vi "Relink Renamed Files to Library.vi"(8 "error in":errorcluster, 10 "plugin library path":path, 11 "plugin files path":path[](array[path])) -> (0 "error out":errorcluster)   [LabVIEW 2021, in "InstrumentStudio Plug-In Editor.lvlib"]
uses:
  InstrumentStudio Plug-In Editor.lvlib
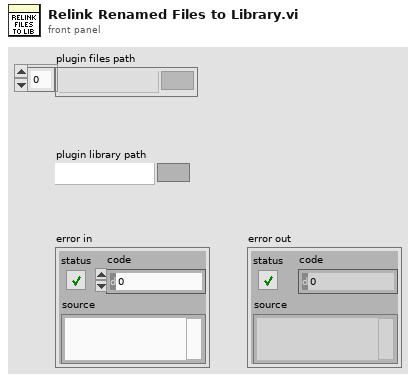
[diagram p1: front panel]
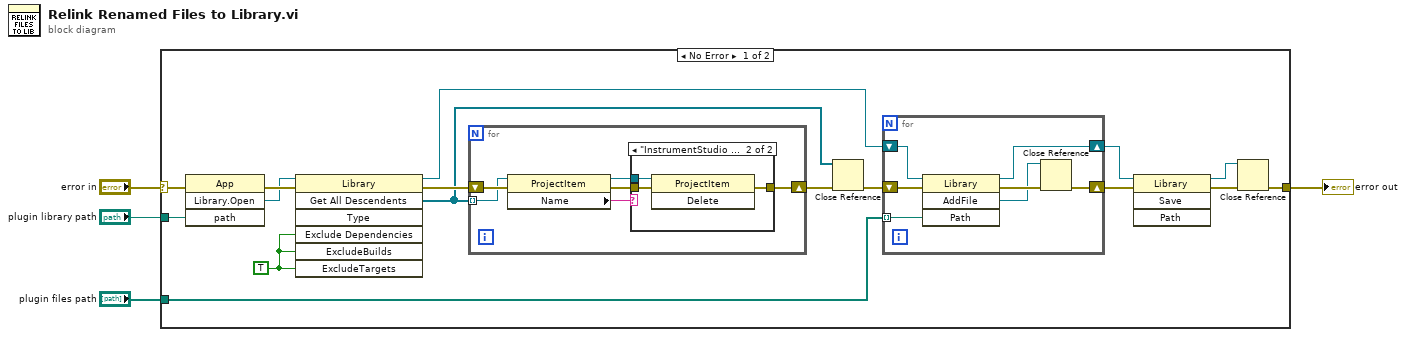
[diagram p0: block diagram]
diagram:
  n1 = case shown="No Error" "error in" {
    selector: "error in" -> [w20 w38]
    tunnel: "plugin library path" -> [w6 _]
    tunnel: [w9 w38] -> w2
    tunnel: "plugin files path" -> [w5 _]
    frame No Error {
      w7 = TRUE ("ExcludeDependencies")
      n2 = invoke class="App" method="Library.Open"(error in=w20, "path"=w6) -> (error out=w19:errorcluster, "Open Library"=w16:refnum<vi>)  [unwired: 2 in, 2 out]
      n3 = invoke class="Library" method="Get All Descendents"(reference=w16, error in=w19, "Exclude Dependencies"=w7, "ExcludeBuilds"=w7, "ExcludeTargets"=w7) -> (reference out=w13:refnum<vi>, error out=w17:errorcluster, "All Descendents"=w8:refnum<vi>[])  [unwired: 2 in, 4 out]
      n4 = for {
        shift-right: [w32] -> w18
        shift-left: w17 -> [w33]
        tunnel: w8 -> [w30] mode=indexing
        n5 = property class="ProjectItem"(reference=w30, error in=w33) -> (reference out=w29:refnum<vi>, error out=w31:errorcluster, "Name"=w28:string)
        n6 = case shown="\"InstrumentStudio Plug-In Template.gplugindata\", \"InstrumentStudio Plug-In Template.vi\"" w28 {
          tunnel: w31 -> [w34 w37]
          tunnel: [w34 w36] -> w32
          tunnel: w29 -> [_ w35]
          frame Default {
          }
          frame "InstrumentStudio Plug-In Template.gplugindata", "InstrumentStudio Plug-In Template.vi" {
            n7 = invoke class="ProjectItem" method="Delete"(reference=w35, error in=w37) -> (error out=w36:errorcluster)  [unwired: 1 in, 2 out]
          }
        }
      }
      n8 = Close Reference(reference=w8, error in (no error)=w18) -> (error out=w15:errorcluster)
      n9 = for {
        shift-right: [w25] -> w14
        shift-left: w15 -> [w27]
        shift-right: [w23] -> w11
        shift-left: w13 -> [w24]
        tunnel: w5 -> [w21] mode=indexing
        n10 = invoke class="Library" method="AddFile"(reference=w24, error in=w27, "Path"=w21) -> (reference out=w23:refnum<vi>, error out=w26:errorcluster, "AddFile"=w22:refnum<vi>)  [unwired: 1 in, 1 out]
        n11 = Close Reference(reference=w22, error in (no error)=w26) -> (error out=w25:errorcluster)
      }
      n12 = invoke class="Library" method="Save"(reference=w11, error in=w14) -> (reference out=w10:refnum<vi>, error out=w12:errorcluster)  [unwired: 2 in, 2 out]
      n13 = Close Reference(reference=w10, error in (no error)=w12) -> (error out=w9:errorcluster)
    }
    frame Error {
    }
  }
  "error out" <- w2
